vi "Excel_Save_Workbook.vi"(0 "Excel._Workbook":refnum<k7>, 5 "password":string, 7 "path":string, 11 "error in (no error)":errorcluster) -> (15 "error out":errorcluster)   [LabVIEW 2010, in "NI_ReportGenerationToolkit.lvlib"]
uses:
  <vilib>/addons/_office/NI_ReportGenerationToolkit.lvlib
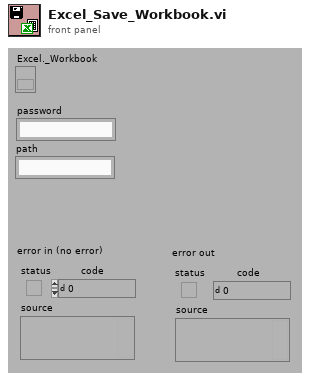
[diagram p1: front panel]
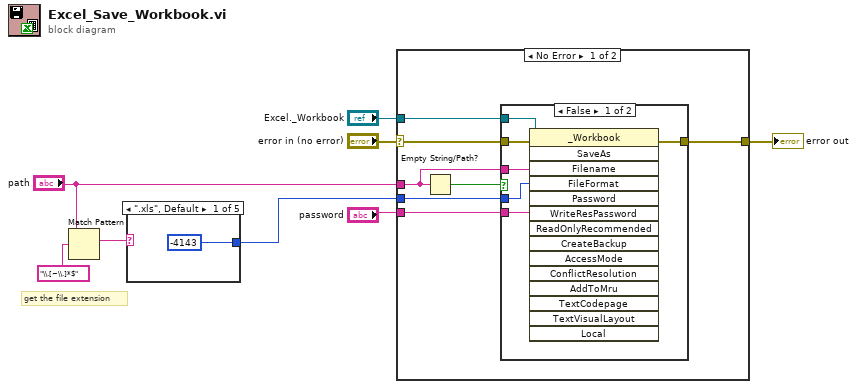
[diagram p0: block diagram]
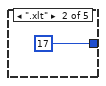
[diagram p2: hidden frame]
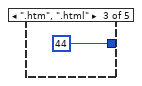
[diagram p3: hidden frame]
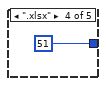
[diagram p4: hidden frame]
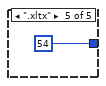
[diagram p5: hidden frame]
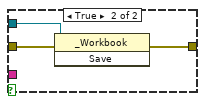
[diagram p6: hidden frame]
diagram:
  # "get the file extension"
  n1 = Match Pattern(string="path", regular expression="\\.[~\\.]*$") -> (match substring=w4:string)  [unwired: 4 out]
  n2 = case shown="\".xls\", Default" w4 {
    tunnel: [-4143 17 44 51 54] -> w1
    frame ".xls", Default {
    }
    frame ".xlt" {
    }
    frame ".htm", ".html" {
    }
    frame ".xlsx" {
    }
    frame ".xltx" {
    }
  }
  n3 = case shown="No Error" "error in (no error)" {
    selector: "error in (no error)" -> [w15 w30]
    tunnel: [w20 w30] -> w8
    tunnel: "Excel._Workbook" -> [w19 _]
    tunnel: "path" -> [w18 _]
    tunnel: "password" -> [w16 _]
    tunnel: w1 -> [w14 _]
    frame No Error {
      n4 = Empty String/Path?(string/path=w18) -> (empty?=w17:bool)
      n5 = case shown="False" w17 {
        tunnel: w19 -> [w24 w29]
        tunnel: w15 -> [w26 w28]
        tunnel: [w25 w27] -> w20
        tunnel: w18 -> [w23 _]
        tunnel: w16 -> [w22 _]
        tunnel: w14 -> [w21 _]
        frame False {
          n6 = invoke class="_Workbook" method="SaveAs"(reference=w24, error in=w26, "Filename"=w23, "FileFormat"=w21, "WriteResPassword"=w22) -> (error out=w25:errorcluster)  [unwired: 10 in, 14 out]
        }
        frame True {
          n7 = invoke class="_Workbook" method="Save"(reference=w29, error in=w28) -> (error out=w27:errorcluster)  [unwired: 1 in, 2 out]
        }
      }
    }
    frame Error {
    }
  }
  "error out" <- w8
